vi "DAQmxTaskContainerFaradayCup-Com-Exec.vi"(8 "error in (no error)":errorcluster, 9 "data":variant, 10 "ControlQueue":refnum<queue>, 11 "DAQmxTaskContainer in":refnum<class "DAQmxTaskContainer.lvclass">) -> (0 "error out":errorcluster, 3 "DAQmxTaskContainer out":refnum<class "DAQmxTaskContainer.lvclass">)   [LabVIEW 2015, in "DAQmxTaskContainer.lvclass"]
uses:
  DAQmxTaskContainer.lvclass
  dependecies/ControlsVIs/Clusters-def/ProtypeCommand-DAQmxReply.ctl
  dependecies/ControlsVIs/Clusters-def/SERVER-Commands.ctl
  dependecies/ControlsVIs/Clusters-def/Message types.ctl
  DAQmxTask.lvclass
  Control/Control-Server/Control-Server.lvclass
  Message/Message.lvclass
  GeneralFunctionality/GeneralFunctionality.lvclass
  DAQmxTaskContainer_General/DAQmxTaksContainer_General.lvclass
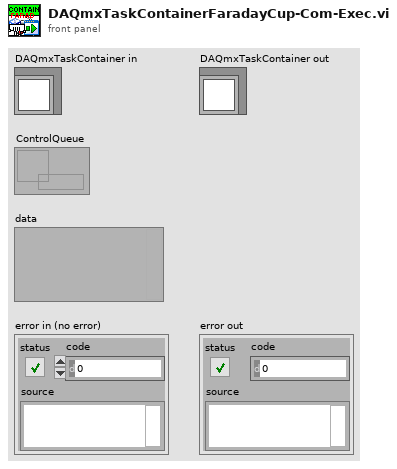
[diagram p1: front panel]
types:
  T1 = typedef "Message types.ctl" = string
  T2 = typedef "Control-Server.lvclass/SERVER-Commands.ctl" = string
  T3 = typedef "ProtypeCommand-DAQmxReply.ctl" = cluster{"On/Off":bool, "error out":errorcluster}
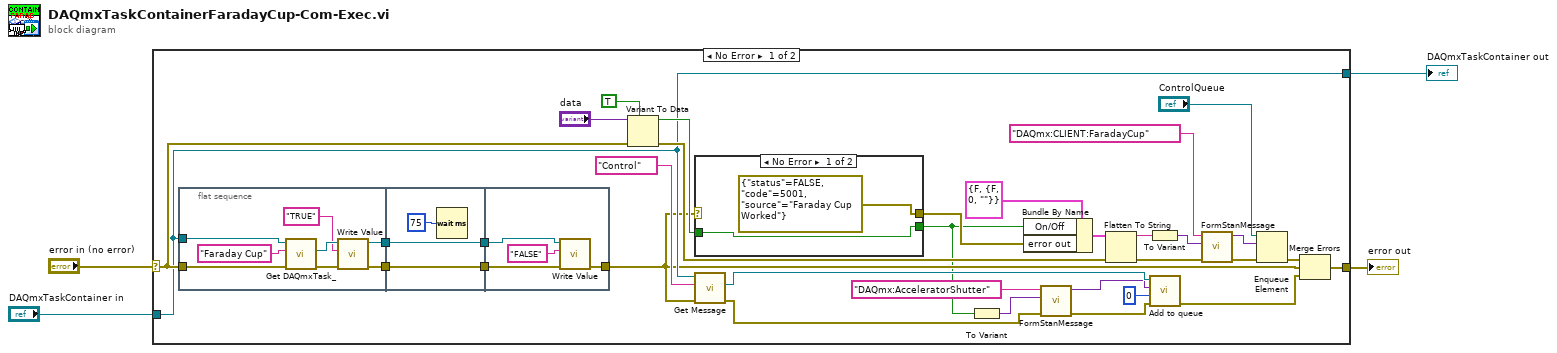
[diagram p0: block diagram]
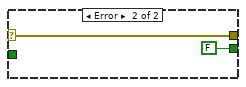
[diagram p2: hidden frame]
diagram:
  n1 = case shown="No Error" "error in (no error)" {
    selector: "error in (no error)" -> [w34 w58]
    tunnel: [w15 w57] -> w4
    tunnel: "DAQmxTaskContainer in" -> [w15 w57]
    tunnel: [w36 w58] -> w2
    frame No Error {
      n2 = flat-sequence {
        tunnel: w15 -> [w45]
        tunnel: w34 -> [w44]
        tunnel: [w39] -> w25
        tunnel: [w38] -> w23
        tunnel: w25 -> [w48]
        tunnel: [w48] -> w24
        tunnel: w23 -> [w46]
        tunnel: [w46] -> w22
        tunnel: [w51] -> w14
        tunnel: w24 -> [w52]
        tunnel: w22 -> [w49]
        frame #0 {
          n3 = call "Get DAQmxTask_.vi"("error in (no error)"=w44, "Task name"="Faraday Cup", "DAQmxTaksContainer_General in"=w45) -> ("error out"=w42:errorcluster, "DAQmx Task"=w41:refnum<class "DAQmxTask.lvclass">)  [unwired: 6 in, 1 out]
          n4 = call-dynamic "Write Value.vi"("error in (no error)"=w42, "Data"="TRUE", "DAQmxTask en entrée"=w41) -> ("error out"=w39:errorcluster, "DAQmxTask en sortie"=w38:refnum<class "DAQmxTask.lvclass">)  [unwired: 7 in]
        }
        frame #1 {
          n5 = Wait (ms)(milliseconds to wait=u32 75) -> ()  [unwired: 1 out]
        }
        frame #2 {
          n6 = call-dynamic "Write Value.vi"("error in (no error)"=w52, "Data"="FALSE", "DAQmxTask en entrée"=w49) -> ("error out"=w51:errorcluster)  [unwired: 7 in, 1 out]
        }
      }
      n7 = Variant To Data(error in=w34, type=TRUE, Variant="data") -> (data=w30:bool, error out=w27:errorcluster)
      n8 = case shown="No Error" w14 {
        selector: w14 -> [_ w56]
        tunnel: [errorcluster {"status"=FALSE, "code"=5001, "source"="Faraday Cup Worked"} ("error constant") w56] -> w31
        tunnel: [w53 FALSE] -> w6
        tunnel: w30 -> [w53 _]
        frame No Error {
        }
        frame Error {
        }
      }
      n9 = call "Get Message.vi"("error in (no error)"=w14, "Message type"=T1 "Control", "GeneralFunctionality en entrée"=w15) -> ("error out"=w12:errorcluster, "Message.lvclass"=w13:refnum<class "Message.lvclass">)  [unwired: 6 in, 1 out]
      n10 = To Variant(anything=w6) -> (Variant=w5:variant)
      n11 = Bundle By Name(cluster=T3 {"On/Off"=FALSE, "error out"={"status"=FALSE, "code"=0, "source"=""}} ("output cluster"), "On/Off"=w6, "error out"=w31) -> (w28:T3)
      n12 = call "FormStanMessage.vi"("error in"=w12, "data"=w5, "Command"="DAQmx:AcceleratorShutter") -> ("error out"=w11:errorcluster, "message"=w10:variant)  [unwired: 7 in]
      n13 = Flatten To String(anything=w28, error in (no error)=w27) -> (data string=w29:string, error out=w19:errorcluster)  [unwired: 2 in, 1 out]
      n14 = To Variant(anything=w29) -> (Variant=w20:variant)
      n15 = call "Add to queue.vi"("error in (no error)"=w11, "timeout in ms (-1)"=0, "Data"=w10, "Message in"=w13) -> ("error out"=w8:errorcluster)  [unwired: 6 in, 1 out]
      n16 = call "FormStanMessage.vi"("error in"=w19, "data"=w20, "Command"=T2 "DAQmx:CLIENT:FaradayCup" ("Commands")) -> ("error out"=w18:errorcluster, "message"=w17:variant)  [unwired: 7 in]
      n17 = Enqueue Element(queue="ControlQueue", element=w17, error in (no error)=w18) -> (error out=w26:errorcluster)  [unwired: 1 in, 2 out]
      n18 = Merge Errors(w26, w14, w8) -> (w36:errorcluster)
    }
    frame Error {
    }
  }
  "DAQmxTaskContainer out" <- w4
  "error out" <- w2
